vi "7.3-ExitPlanningEventHandler.vi"() -> (0 "Main Tab Interface  2":T1, 1 "T button?":bool)   [LabVIEW 2010]
uses:
  TabEnum.ctl
  7.0-Global.vi
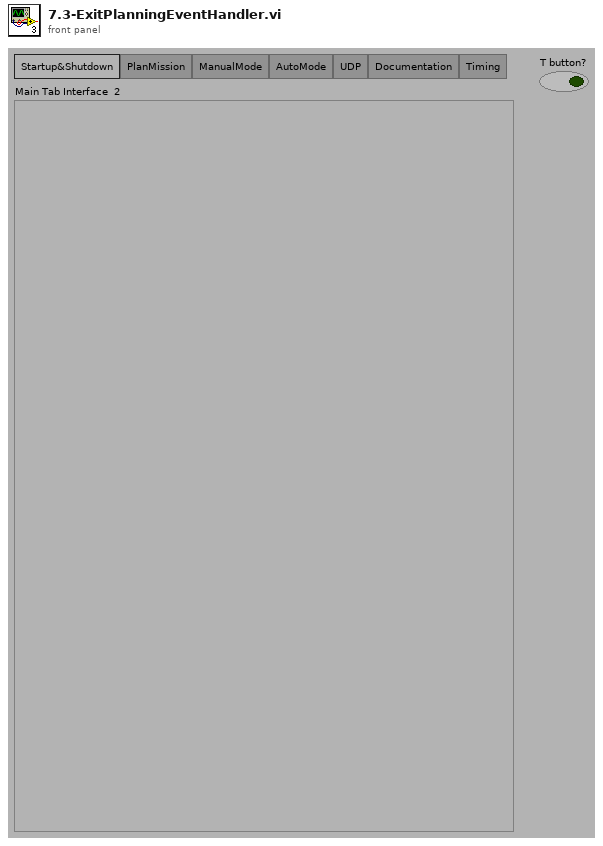
[diagram p1: front panel]
types:
  T1 = typedef "TabEnum.ctl" = enum32{"Startup&Shutdown", "PlanMission", "ManualMode", "AutoMode", "UDP", "Documentation", "Timing"}
  T2 = enum32{"7.1-Act", "7.2-Where", "7.3-What", "7.4-How", "Startup&Shutdown", "PlanMission", "ManualMode", "AutoMode", "UDP", "Documentation", "7.8-Timing"}
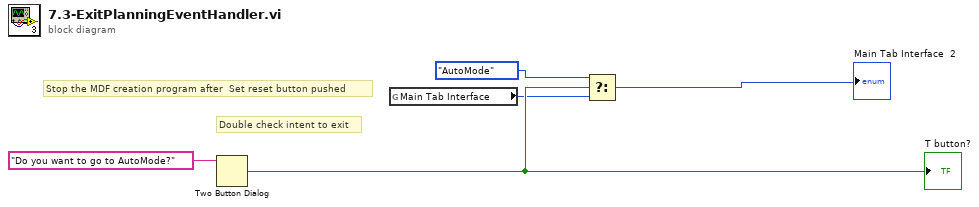
[diagram p0: block diagram]
diagram:
  # "Double check intent to exit"
  # "Stop the MDF creation program after  Set reset button pushed"
  n1 = Two Button Dialog(message="Do you want to go to AutoMode?") -> (T button?=w4:bool)  [unwired: 2 in]
  "T button?" <- w4
  n2 = global read "7.0-Global.vi" "Main Tab Interface"() -> (w2:T2)
  n3 = Select(t=TabEnum."AutoMode" ("Main Tab Interface  2"), s=w4, f=w2) -> (s? t:f=→"Main Tab Interface  2":u32)
